vi "Set_J17Low-J18High.vi"(3 "error in":errorcluster) -> (10 "error out":errorcluster)   [LabVIEW 2015]
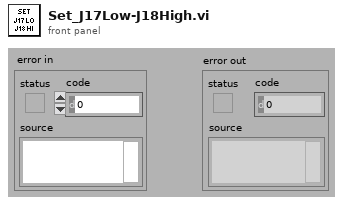
[diagram p1: front panel]
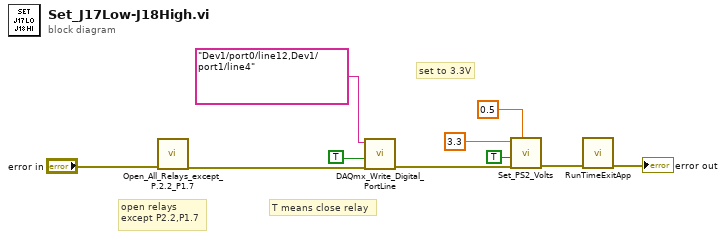
[diagram p0: block diagram]
diagram:
  # "open relays\nexcept P2.2,P1.7"
  # "T means close relay"
  # "set to 3.3V"
  n1 = call "Open_All_Relays_except_P.2.2_P1.7.vi"("error in"="error in") -> ("error out"=w1:errorcluster)  [unwired: 8 in]
  n2 = call "DAQmx_Write_Digital_PortLine.vi"("Device/Ports/Lines"="Dev1/port0/line12,Dev1/port1/line4", "Boolean"=TRUE, "error in"=w1) -> ("error out"=w8:errorcluster)  [unwired: 6 in, 1 out]
  n3 = call "Set_PS2_Volts.vi"("delay (secs)"=0.5, "error in"=w8, "Output on/off"=TRUE, "Output Voltage"=3.3 ("Output Voltage (0)")) -> ("error out"=w7:errorcluster)  [unwired: 5 in, 2 out]
  n4 = call "RunTimeExitApp.vi"("error in (no error)"=w7) -> ("error out"=→"error out":errorcluster)  [unwired: 10 in]
